vi "readinRfXML.vi"(8 "error in (no error)":errorcluster, 10 "xml in":refnum<class "NativeXML.lvclass">, 11 "deviceDataBase in":refnum<class "deviceDataBase.lvclass">) -> (0 "error out":errorcluster, 2 "device.lvclass out":refnum<class "device.lvclass">, 3 "deviceDataBase out":refnum<class "deviceDataBase.lvclass">)   [LabVIEW 2011, in "Tools.lvlib" / "DatabaseHelpers.lvlib" / "deviceDataBase.lvclass"]
uses:
  deviceDataBase.lvclass
  NativeXML/NativeXML.lvclass
  Database Objects/device/device.lvclass
  Database Objects/device/rfDevice/rfDevice.lvclass
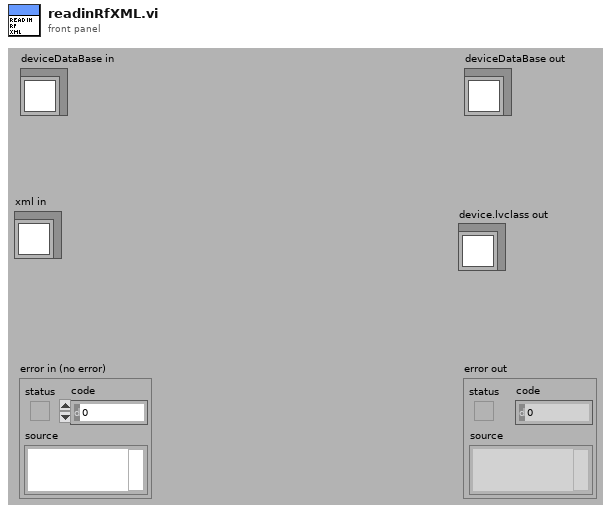
[diagram p1: front panel]
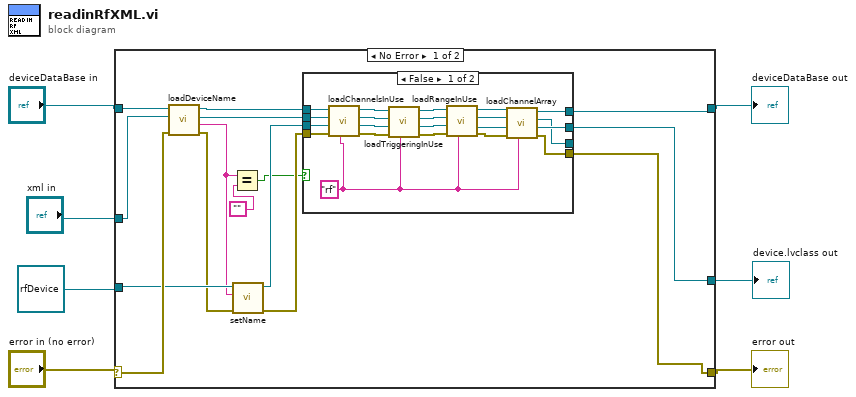
[diagram p0: block diagram]
diagram:
  n1 = case shown="No Error" "error in (no error)" {
    selector: "error in (no error)" -> [w21 w49]
    tunnel: [w8 w49] -> w2
    tunnel: [w12 w48] -> w7
    tunnel: "deviceDataBase in" -> [w22 w48]
    tunnel: "xml in" -> [w20 _]
    tunnel: refnum<class "rfDevice.lvclass"> refnum ("Tools.lvlib:DatabaseHelpers.lvlib:rfDevice.lvclass") -> [w19 _]
    tunnel: [w13 _] -> w1
    frame No Error {
      n2 = call "loadDeviceName.vi"("error in (no error)"=w21, "NativeXML in"=w20, "deviceDataBase in"=w22) -> ("error out"=w18:errorcluster, "deviceName"=w10:string, "NativeXML out"=w15:refnum<class "NativeXML.lvclass">, "deviceDataBase out"=w17:refnum<class "deviceDataBase.lvclass">)  [unwired: 5 in]
      n3 = Equal?(x=w10, y="") -> (x = y?=w11:bool)
      n4 = call "setName.vi"("error in (no error)"=w18, "name"=w10, "device.lvclass in"=w19) -> ("error out"=w16:errorcluster, "device.lvclass out"=w14:refnum<class "rfDevice.lvclass">)  [unwired: 7 in]
      n5 = case shown="False" w11 {
        tunnel: w17 -> [w43 w47]
        tunnel: w16 -> [w42 w45]
        tunnel: w15 -> [w41 w44]
        tunnel: w14 -> [w40 w46]
        tunnel: [w27 w45] -> w8
        tunnel: [w26 w46] -> w13
        tunnel: [w25 w47] -> w12
        tunnel: [w24 w44] -> _
        frame False {
          w23 = "rf"
          n6 = call "loadChannelsInUse.vi"("type"=w23, "error in (no error)"=w42, "device.lvclass"=w40, "NativeXML in"=w41, "deviceDataBase in"=w43) -> ("error out"=w39:errorcluster, "device.lvclass out"=w36:refnum<class "device.lvclass">, "NativeXML out"=w37:refnum<class "NativeXML.lvclass">, "deviceDataBase out"=w38:refnum<class "deviceDataBase.lvclass">)  [unwired: 3 in]
          n7 = call "loadTriggeringInUse.vi"("type"=w23, "error in (no error)"=w39, "device.lvclass"=w36, "NativeXML in"=w37, "deviceDataBase in"=w38) -> ("error out"=w32:errorcluster, "device.lvclass out"=w33:refnum<class "device.lvclass">, "NativeXML out"=w34:refnum<class "NativeXML.lvclass">, "deviceDataBase out"=w35:refnum<class "deviceDataBase.lvclass">)  [unwired: 3 in]
          n8 = call "loadRangeInUse.vi"("type"=w23, "error in (no error)"=w32, "device.lvclass"=w33, "NativeXML in"=w34, "deviceDataBase in"=w35) -> ("error out"=w30:errorcluster, "device.lvclass out"=w28:refnum<class "device.lvclass">, "NativeXML out"=w29:refnum<class "NativeXML.lvclass">, "deviceDataBase out"=w31:refnum<class "deviceDataBase.lvclass">)  [unwired: 3 in]
          n9 = call "loadChannelArray.vi"("type"=w23, "error in (no error)"=w30, "device.lvclass"=w28, "NativeXML in"=w29, "deviceDataBase in"=w31) -> ("error out"=w27:errorcluster, "device.lvclass out"=w26:refnum<class "device.lvclass">, "NativeXML out"=w24:refnum<class "NativeXML.lvclass">, "deviceDataBase out"=w25:refnum<class "deviceDataBase.lvclass">)  [unwired: 3 in]
        }
        frame True {
        }
      }
    }
    frame Error {
    }
  }
  "error out" <- w2
  "deviceDataBase out" <- w7
  "device.lvclass out" <- w1
